vi "Coord window-PictureMap menu handler.vi"(11 "ItemTag":string) -> ()   [LabVIEW 2020]
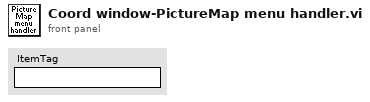
[diagram p1: front panel]
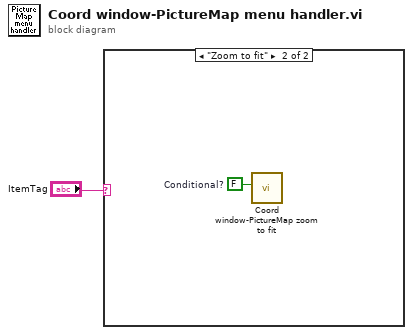
[diagram p0: block diagram]
diagram:
  n1 = case shown="\"Zoom to fit\"" "ItemTag" {
    frame Default {
    }
    frame "Zoom to fit" {
      w2 = FALSE  # Conditional?
      n2 = call "Coord window-PictureMap zoom to fit.vi"("Conditional?"=w2) -> ()  [unwired: 10 in, 1 out]
    }
  }
